vi "Read Displayed Seconds on Timing.vi"(8 "error in (no error)":errorcluster, 11 "Configuration Database in":refnum<class "Configuration Database.lvclass">) -> (0 "error out":errorcluster, 2 "Time(Sec)":dbl, 3 "Configuration Database out":refnum<class "Configuration Database.lvclass">)   [LabVIEW 2019, in "Configuration Database Actor.lvlib" / "Configuration Database.lvclass"]
uses:
  Configuration Database.lvclass
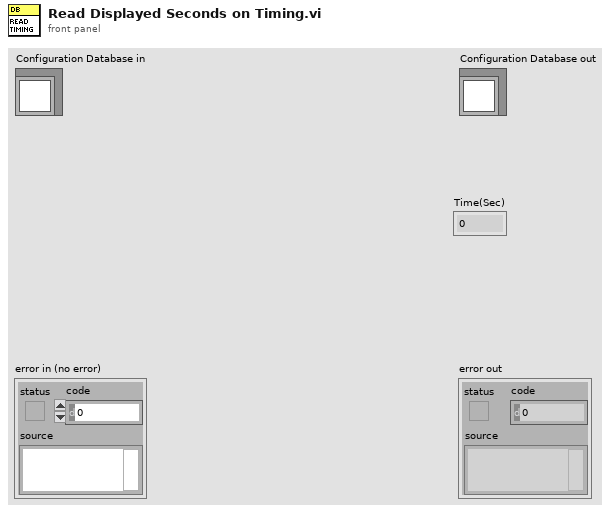
[diagram p1: front panel]
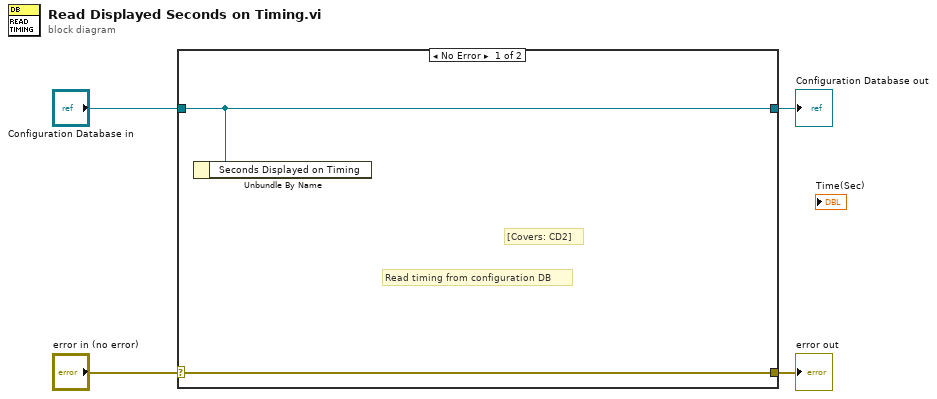
[diagram p0: block diagram]
diagram:
  n1 = case shown="No Error" "error in (no error)" {
    selector: "error in (no error)" -> [w6 w8]
    tunnel: [w6 w8] -> w3
    tunnel: [w5 w7] -> w1
    tunnel: "Configuration Database in" -> [w5 w7]
    frame No Error {
      # "[Covers: CD2]"
      # "Read timing from configuration DB"
      n2 = Unbundle By Name(w5) -> ()  [unwired: 1 out]
    }
    frame Error {
    }
  }
  "error out" <- w3
  "Configuration Database out" <- w1
